vi "E7_30_write.vi"(5 "VALUE":T7, 7 "Command":T7, 8 "error in":T8, 11 "DriverConnect in":T1={"InterfaceType"=enum."VISA", "OpenedSession"="", "InterfaceSettings"={"Interface"=enum."RS232", "EOS 4 read"=enum."LF (\\n)", "EOS 4 write"=enum."LF (\\n)", "TMO, ms"=10000, "Sett"=variant(cluster{"Baud Rate":u32, "Data Bits":u16, "Parity":u16, "Stop Bits":u16, "Flow Control":u16, "Eho":bool} {"Baud Rate"=75, "Data Bits"=0, "Parity"=0, "Stop Bits"=0, "Flow Control"=0, "Eho"=FALSE})}}) -> (0 "error out":T8, 3 "DriverConnect out":T1={"InterfaceType"=enum."VISA", "OpenedSession"="", "InterfaceSettings"={"Interface"=enum."RS232", "EOS 4 read"=enum."LF (\\n)", "EOS 4 write"=enum."LF (\\n)", "TMO, ms"=10000, "Sett"=variant(cluster{"Baud Rate":u32, "Data Bits":u16, "Parity":u16, "Stop Bits":u16, "Flow Control":u16, "Eho":bool} {"Baud Rate"=75, "Data Bits"=0, "Parity"=0, "Stop Bits"=0, "Flow Control"=0, "Eho"=FALSE})}}, 4 "command HEX out":T6, 6 "command string out":T7)   [LabVIEW 2018]
uses:
  MOKO_LabViewLibrary/MokoLowLevel/MokoLowLovelControl/MLLC_Error.ctl
  MOKO_LabViewLibrary/MokoLowLevel/MokoLowLovelControl/MLLC_Command.ctl
  MOKO_LabViewLibrary/MokoLowLevel/MokoLowLovelControl/MLLC_ErrorCode.ctl
  MOKO_LabViewLibrary/MokoLowLevel/MokoLowLovelControl/MLLC_ConnectCluster.ctl
  MOKO_LabViewLibrary/MokoLowLevel/MokoLowLovelControl/MLLC_InterfaceType.ctl
  MOKO_LabViewLibrary/MokoLowLevel/MokoLowLovelControl/MLLC_OpenedSession.ctl
  MOKO_LabViewLibrary/MokoLowLevel/MokoLowLovelControl/MLLC_InterfaceSettings.ctl
  MOKO_LabViewLibrary/MokoLowLevel/MokoLowLovelControl/MLLC_InterfaceKind.ctl
panel:
  out "Message Based Settings:Termination Character":T6
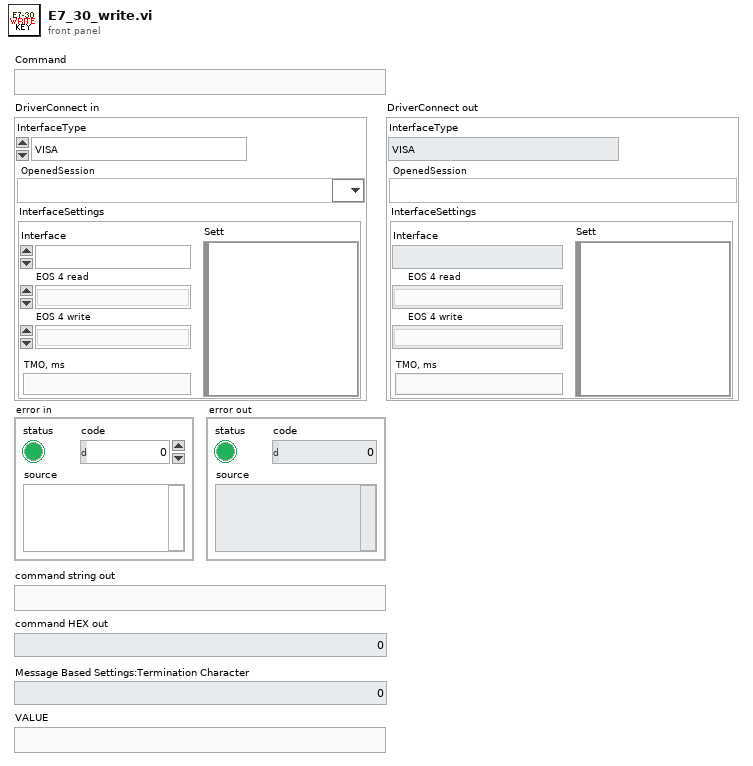
[diagram p1: front panel]
types:
  T1 = typedef "MLLC_ConnectCluster.ctl" = cluster{"InterfaceType":T2, "OpenedSession":T3, "InterfaceSettings":T4}
  T2 = typedef "MLLC_InterfaceType.ctl" = enum16{"VISA", "Prologix USB-GPIB"}
  T3 = typedef "MLLC_OpenedSession.ctl" = refnum<visa-resource-name>
  T4 = typedef "MLLC_InterfaceSettings.ctl" = cluster{"Interface":T5, "EOS 4 read":enum16{"Default (=EOS 4 write)", "CR (\\r)", "LF (\\n)", "None"}, "EOS 4 write":enum16{"CR+LF (\\r\\n)", "CR (\\r)", "LF (\\n)", "None"}, "TMO, ms":i32, "Sett":variant}
  T5 = typedef "MLLC_InterfaceKind.ctl" = enum16{"RS232", "GPIB", "USB", "Ethernet", "another"}
  T6 = typedef "MLLC_ErrorCode.ctl" = u32
  T7 = typedef "MLLC_Command.ctl" = string
  T8 = typedef "MLLC_Error.ctl" = errorcluster
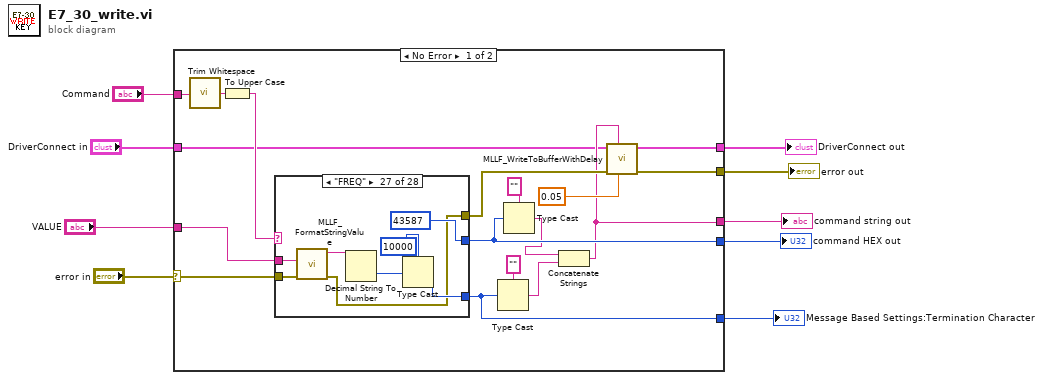
[diagram p0: block diagram]
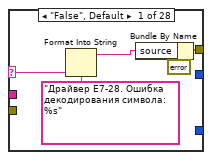
[diagram p2: hidden frame]
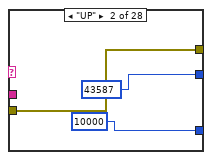
[diagram p3: hidden frame]
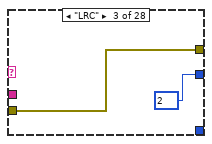
[diagram p4: hidden frame]
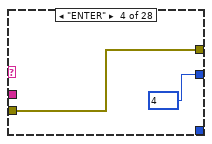
[diagram p5: hidden frame]
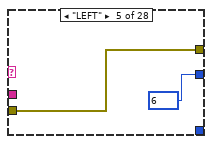
[diagram p6: hidden frame]
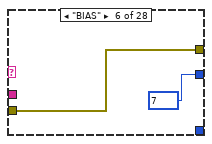
[diagram p7: hidden frame]
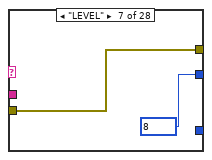
[diagram p8: hidden frame]
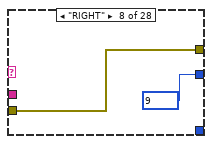
[diagram p9: hidden frame]
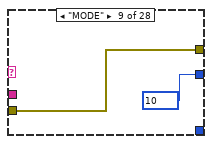
[diagram p10: hidden frame]
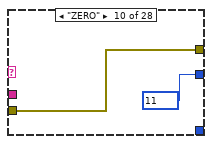
[diagram p11: hidden frame]
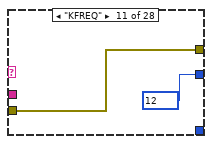
[diagram p12: hidden frame]
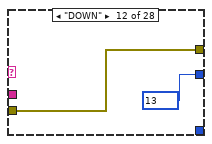
[diagram p13: hidden frame]
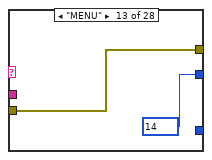
[diagram p14: hidden frame]
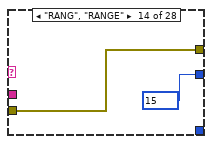
[diagram p15: hidden frame]
diagram:
  n1 = case shown="No Error" "error in" {
    selector: "error in" -> [w11 w72]
    tunnel: [w20 w72] -> w9
    tunnel: [w21 w71] -> w1
    tunnel: "Command" -> [w23 _]
    tunnel: [w16 _] -> w6
    tunnel: [w19 _] -> w5
    tunnel: "VALUE" -> [w12 _]
    tunnel: [w13 _] -> w3
    tunnel: "DriverConnect in" -> [w10 w71]
    frame No Error {
      n2 = call <vilib>:"Trim Whitespace.vi"("string"=w23) -> ("trimmed string"=w24:string)  [unwired: 1 in]
      n3 = To Upper Case(1:w24) -> (0:w22:string)
      n4 = case shown="\"FREQ\"" w22 {
        selector: w22 -> [w28 _ _ _ _ _ _ _ _ _ _ _ _ _ _ _ _ _ _ _ _ _ _ _ _ _ _ _]
        tunnel: [w30 w34 w36 w38 w40 w42 w44 w46 w48 w50 w52 w54 w56 w58 _ _ _ _ _ _ _ _ _ _ w59 w61 w63 _] -> w26
        tunnel: w11 -> [_ w34 w36 w38 w40 w42 w44 w46 w48 w50 w52 w54 w56 w58 _ _ _ _ _ _ _ _ _ _ w59 w61 w64 _]
        tunnel: [_ u16 43587 ("Message Based Settings:Termination Character") u16 2 ("length (rest)") u16 4 ("length (rest)") u16 6 ("length (rest)") u16 7 ("length (rest)") u16 8 ("length (rest)") u16 9 ("length (rest)") u16 10 ("length (rest)") u16 11 ("length (rest)") u16 12 ("length (rest)") u16 13 ("length (rest)") u16 14 ("length (rest)") u16 15 ("length (rest)") _ _ _ _ _ _ _ _ _ _ u16 43584 ("Message Based Settings:Termination Character") u16 43592 ("Message Based Settings:Termination Character") u16 43587 ("Message Based Settings:Termination Character") _] -> w19
        tunnel: w12 -> [_ _ _ _ _ _ _ _ _ _ _ _ _ _ _ _ _ _ _ _ _ _ _ _ _ _ w66 _]
        tunnel: [_ u32 10000 ("Message Based Settings:Termination Character") _ _ _ _ _ _ _ _ _ _ _ _ _ _ _ _ _ _ _ _ _ _ _ _ w68 _] -> w13
        frame "False", Default {
          n5 = Format Into String(format string="Драйвер Е7-28. Ошибка декодирования символа: %s" ("source"), w28) -> (resulting string=w29:string)  [unwired: 2 in, 1 out]
          n6 = Bundle By Name(cluster=errorcluster {"status"=TRUE, "code"=5436, "source"="Драйвер Г5-82. Ошибка декодирования символа: %s"} ("error IO"), "source"=w29) -> (w30:errorcluster)
        }
        frame "UP" {
        }
        frame "LRC" {
        }
        frame "ENTER" {
        }
        frame "LEFT" {
        }
        frame "BIAS" {
        }
        frame "LEVEL" {
        }
        frame "RIGHT" {
        }
        frame "MODE" {
        }
        frame "ZERO" {
        }
        frame "KFREQ" {
        }
        frame "DOWN" {
        }
        frame "MENU" {
        }
        frame "RANG", "RANGE" {
        }
        frame "17" {
        }
        frame "18" {
        }
        frame "19" {
        }
        frame "20" {
        }
        frame "21" {
        }
        frame "22" {
        }
        frame "24" {
        }
        frame "25" {
        }
        frame "26" {
        }
        frame "27" {
        }
        frame "INIT" {
          # "инициализация"
        }
        frame "READ" {
          # "считать параметры"
        }
        frame "FREQ" {
          n7 = call "MLLF_FormatStringValue.vi"("error in"=w64, "String Value"=w66) -> ("error out"=w63:T8, "String Value Formated"=w65:T7)  [unwired: 7 in, 1 out]
          n8 = Decimal String To Number(string=w65) -> (number=w67:i32)  [unwired: 2 in, 1 out]
          n9 = Type Cast(type=u32 10000 ("Message Based Settings:Termination Character"), x=w67) -> (*(type *) &x=w68:u32)
        }
        frame "AVP" {
        }
      }
      n10 = Type Cast(type="", x=w13) -> (*(type *) &x=w14:string)
      n11 = Type Cast(type="", x=w19) -> (*(type *) &x=w17:string)
      n12 = Concatenate Strings(w17, w14) -> (w16:string)
      n13 = call "MLLF_WriteToBufferWithDelay.vi"("Delay Time ( 0,05 s)"=0.05 ("Delay Time (s)"), "Command"=w16, "Error In"=w26, "DriverConnect in"=w10) -> ("Error Out"=w20:errorcluster, "DriverConnect out"=w21:T1)  [unwired: 6 in]
    }
    frame Error {
    }
  }
  "error out" <- w9
  "command string out" <- w6
  "command HEX out" <- w5
  "Message Based Settings:Termination Character" <- w3
  "DriverConnect out" <- w1
